vi "ExSubROIBin2xSameDim.vi"(2 "error in (no error)":errorcluster, 3 "Camera Handle":u32) -> (0 "error out":errorcluster, 1 "Camera Handle":u32)   [LabVIEW 2010]
panel:
  # "ExSubROIBin2xSameDim:\nThis Sub-VI bins chip by 2 in both x \nand y dimensions. It also make sure \nthe final result is the same. This is \nso we don't run into any problems \nwith the Rotate example."
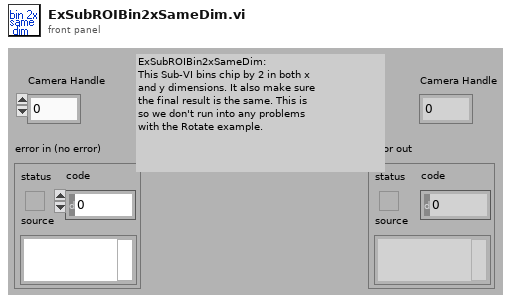
[diagram p1: front panel]
types:
  T1 = cluster{"X start":u32, "X end":u32, "X Binning/Grouping":u32, "Y start":u32, "Y end":u32, "Y Binning/Grouping":u32}
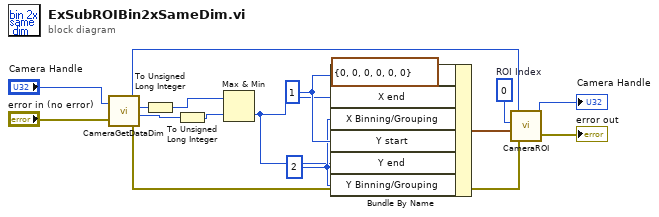
[diagram p0: block diagram]
diagram:
  w9 = u32 0  # ROI Index
  w7 = u32 2
  w8 = u32 1
  n1 = call <userlib>:"CameraGetDataDim.vi"("Camera Handle"="Camera Handle", "error in"="error in (no error)") -> ("Camera Handle"=w15:u32, "Xdim"=w6:u32, "Ydim"=w5:u32, "error out"=w13:errorcluster)
  n2 = To Unsigned Long Integer(number=w6) -> (unsigned 32bit integer=w3:u32)
  n3 = To Unsigned Long Integer(number=w5) -> (unsigned 32bit integer=w2:u32)
  n4 = Max & Min(x=w3, y=w2) -> (min(x,y)=w1:u32)  [unwired: 1 out]
  n5 = Bundle By Name(cluster=T1 {"X start"=0, "X end"=0, "X Binning/Grouping"=0, "Y start"=0, "Y end"=0, "Y Binning/Grouping"=0} ("ROI Params"), "X start"=w8, "X end"=w1, "X Binning/Grouping"=w7, "Y start"=w8, "Y end"=w1, "Y Binning/Grouping"=w7) -> (w4:T1)
  n6 = call <userlib>:"CameraROI.vi"("error in"=w13, "ROI Params"=w4, "ROI Index"=w9, "Camera Handle"=w15) -> ("error out"=→"error out":errorcluster, "Camera Handle"=→"Camera Handle":u32)
